vi "LoadVisionValues.vi"(8 "error in":errorcluster) -> (0 "error out":errorcluster)   [LabVIEW 2015]
uses:
  Vision/Camera Settings Type Def.ctl
  <vilib>/Rock Robotics/WPI/Camera/WPI_CameraWhite Balance Values.ctl
  <vilib>/Rock Robotics/WPI/Camera/WPI_CameraExposure Values.ctl
  <vilib>/Rock Robotics/Network Tables/NT Read Numeric Array.vi
  Vision/Vision Global.vi
panel:
  out "Settings":T1={"FPS"=0.0, "White Balance"=enum."Fixed indoor", "Exposure"=enum."Flicker-free 60 Hz", "Compression"=0.0, "Brightness"=0.0}
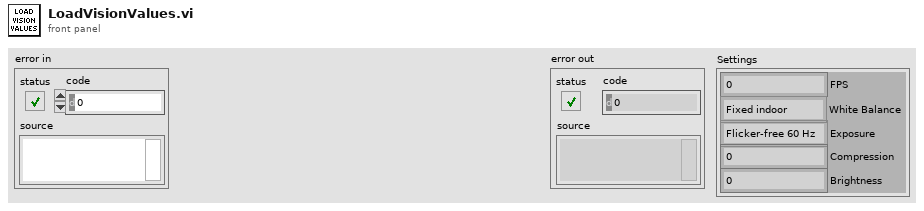
[diagram p1: front panel]
types:
  T1 = typedef "Camera Settings Type Def.ctl" = cluster{"FPS":dbl, "White Balance":T2, "Exposure":T3, "Compression":dbl, "Brightness":dbl}
  T2 = typedef "WPI_CameraWhite Balance Values.ctl" = enum16{"Auto", "Fixed indoor", "Fixed outdoor 1", "Fixed outdoor 2", "Fixed fluorescent 1", "Fixed fluorescent 2", "Hold current", "Custom"}
  T3 = typedef "WPI_CameraExposure Values.ctl" = enum16{"Auto", "Flicker-free 50 Hz", "Flicker-free 60 Hz", "Hold current", "Custom"}
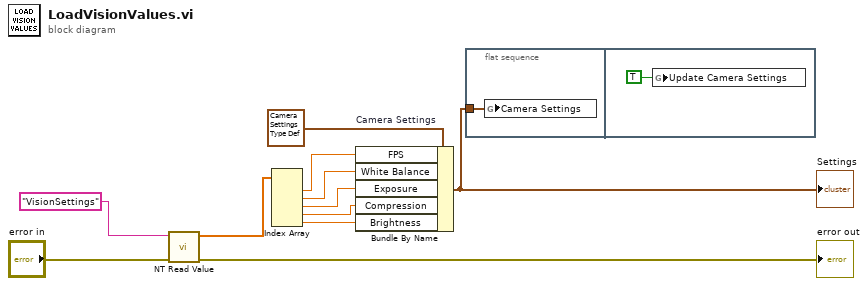
[diagram p0: block diagram]
diagram:
  n1 = call-poly <vilib>:"NT Read Value.vi"("error in"="error in", "Name"="VisionSettings") -> ("error out"=→"error out":errorcluster, "Numeric Array"=w4:dbl[])  [unwired: 8 in]
  n2 = Index Array(array=w4) -> (element #1=w6:dbl, element #2=w7:dbl, element #3=w8:dbl, element #4=w9:dbl, element #5=w10:dbl)  [unwired: 5 in]
  n3 = Bundle By Name "Camera Settings"(cluster=T1 {"FPS"=0.0, "White Balance"=enum."Fixed indoor", "Exposure"=enum."Flicker-free 60 Hz", "Compression"=0.0, "Brightness"=0.0} ("Camera Settings"), "FPS"=w6, "White Balance"=w7, "Exposure"=w8, "Compression"=w9, "Brightness"=w10) -> (w11:T1)
  "Settings" <- w11
  n4 = flat-sequence {
    tunnel: w11 -> [w12]
    frame #0 {
      n5 = global write "Vision Global.vi" "Camera Settings"(w12) -> ()
    }
    frame #1 {
      n6 = global write "Vision Global.vi" "Update Camera Settings"(TRUE ("Update Camera Settings")) -> ()
    }
  }
